vi "Hokuyo initialize.vi"(3 "real/sim":bool, 4 "Hokuyo Port":refnum<visa-resource-name>="COM15") -> (1 "LMS Information Cluster":T1)   [LabVIEW 2014]
uses:
  Initialize-Standard.vi
  Hokuyo URG Series.lvlib
panel:
  in  "Reset?":bool=TRUE
  in  "Magnitude":dbl[](array[numeric])
  in  "LMS Local Map":i32[][](array[numeric])
  in  "Protocol":u32(ring)=2 items=["Convert to Latest", "SCIP 1.1", "SCIP 2.0"]
  in  "ID Query?":bool=TRUE
  in  "Checksum":bool
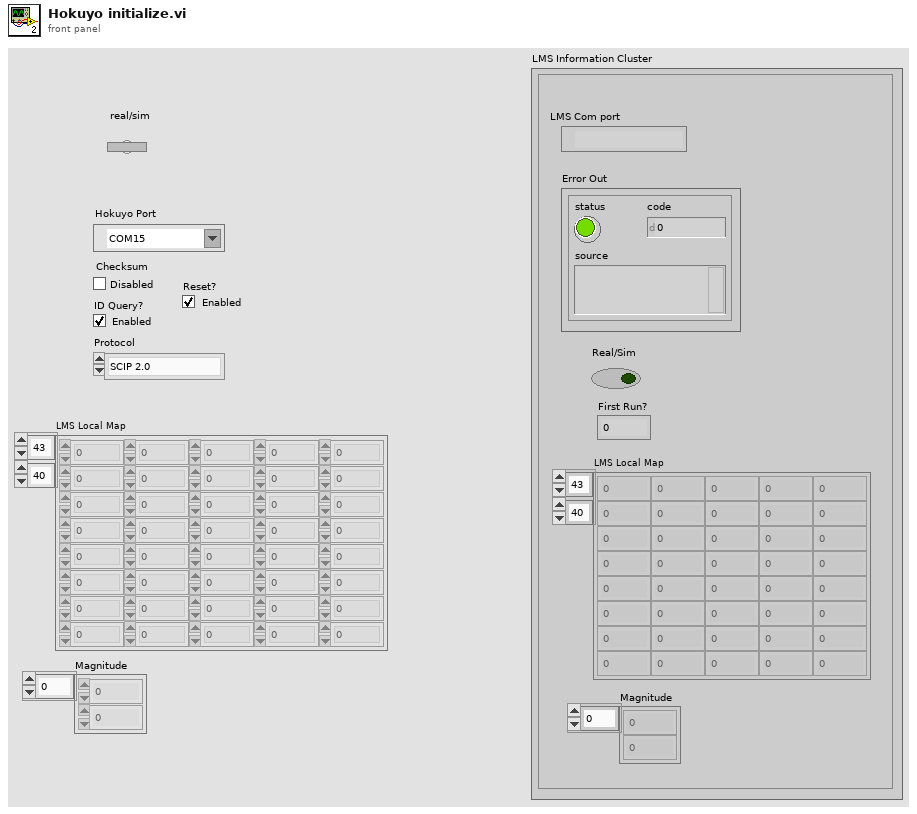
[diagram p1: front panel]
types:
  T1 = cluster{"LMS Com port":refnum<visa-resource-name>, "Error Out":errorcluster, "Real/Sim":bool, "First Run?":i32, "LMS Local Map ":dbl[][], "Magnitude":dbl[]}
  T2 = cluster{"VISA resource name out":refnum<visa-resource-name>, "error out":errorcluster, "real/sim\n":bool, "Numeric":i32, "LMS Local Map ":i32[][], "Magnitude":dbl[]}
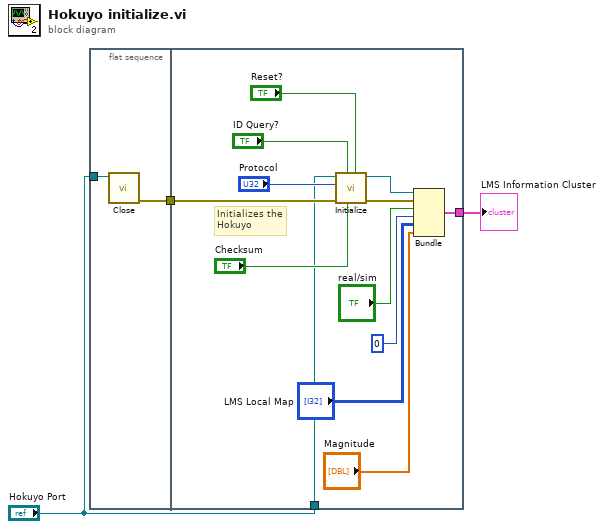
[diagram p0: block diagram]
diagram:
  n1 = flat-sequence {
    tunnel: "Hokuyo Port" -> [w5]
    tunnel: [w4] -> w2
    tunnel: [w12] -> w3
    tunnel: w2 -> [w7]
    tunnel: "Hokuyo Port" -> [w6]
    frame #0 {
      n2 = call "Close.vi"("VISA resource name"=w5) -> ("error out"=w4:errorcluster)  [unwired: 10 in]
    }
    frame #1 {
      # "Initializes the Hokuyo"
      n3 = call-poly "Initialize.vi"("Reset? (F: No)"="Reset?", "Checksum (Disabled)"="Checksum", "ID Query? (Enabled)"="ID Query?", "error in (no error)"=w7, "Protocol (2: SCIP 2.0)"="Protocol", "VISA resource name"=w6) -> ("error out"=w14:errorcluster, "VISA resource name out"=w15:refnum<visa-resource-name>)  [unwired: 4 in]
      n4 = Bundle("VISA resource name out"=w15, "error out"=w14, "real/sim"="real/sim", "Numeric"=0, "LMS Local Map"="LMS Local Map", "Magnitude"="Magnitude") -> (w12:T2)  [unwired: 1 in]
    }
  }
  "LMS Information Cluster" <- w3
